vi "WPI_DashboardListFiles.vi"(11 "Path":path) -> (3 "FileNames":string[](array[string]))   [LabVIEW 2019]
doc: "Returns the list of Dashboard recoreding files from the specified location. If not wired, it uses the typical location for dashboard storage."
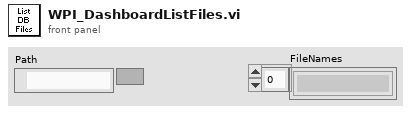
[diagram p1: front panel]
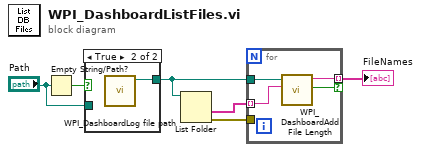
[diagram p0: block diagram]
diagram:
  n1 = Empty String/Path?(string/path="Path") -> (empty?=w2:bool)
  n2 = case shown="True" w2 {
    tunnel: [w7 w8] -> w6
    tunnel: "Path" -> [w7 _]
    frame False {
    }
    frame True {
      n3 = call <vilib>:"WPI_DashboardLog file path.vi"() -> ("appended path"=w8:path)  [unwired: 11 in]
    }
  }
  n4 = List Folder(path=w6) -> (folder names=w4:string[], error out=w5:errorcluster)  [unwired: 3 in, 2 out]
  n5 = for {
    tunnel: w4 -> [w10] mode=indexing
    tunnel: [w12] -> w3 mode=indexing if=w9
    tunnel: w6 -> [w11]
    tunnel: w5 -> [_]
    n6 = call <vilib>:"WPI_DashboardAdd File Length.vi"("String in"=w10, "appended path"=w11) -> ("Valid"=w9:bool, "String out"=w12:string)  [unwired: 8 in]
  }
  "FileNames" <- w3
